vi "Register for gRPC Server Events.vi"(8 "error in (no error)":errorcluster, 11 "Plugin Manager in":refnum<class "CIFPluginManager.lvclass">) -> (0 "error out":errorcluster, 2 "Event Registration Refnum":refnum<event-registration>, 3 "Plugin Manager out":refnum<class "CIFPluginManager.lvclass">)   [LabVIEW 2021, in "CIFPluginManager.lvclass"]
uses:
  CIFPluginManager.lvclass
  CIF_Manager_server/RPC Service/Manager/Manager.lvclass
  C:/Program Files/National Instruments/LabVIEW 2021/vi.lib/gRPC/LabVIEW gRPC Servicer/ServiceBase/ServiceBase.lvclass
  CIF_Manager_server/RPC Service/Manager/Manager.lvclass/Manager.ctl
  CIFPluginManager.lvclass/CIFPluginManager.ctl
  D:/dev/CIF-LVCore/src/CIFPluginManager/CIFPluginManager/gRPC/CIF_Manager_server/RPC Service/Manager/Manager.lvclass
  <vilib>/gRPC/LabVIEW gRPC Library/Shared/grpcId.ctl
  <vilib>/gRPC/LabVIEW gRPC Library/grpc-lvsupport-release.lvlib
  <vilib>/gRPC/LabVIEW gRPC Library/Server API/typeDefs/gRPCId Cluster.ctl
  CIF_Manager_server/RPC Service/Manager/typeDefs/Server gRPC UEs.ctl
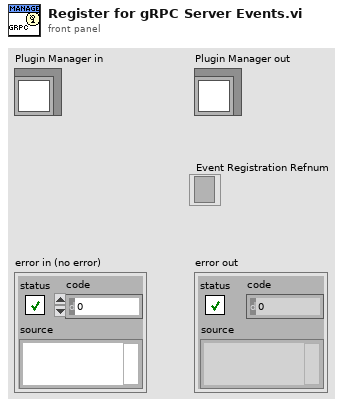
[diagram p1: front panel]
types:
  T1 = typedef "CIF_Manager_server.lvlib/Manager.lvclass/Server gRPC UEs.ctl" = cluster{"Manager LoadPlugin gRPC UE":refnum<user-event>, "Manager RegisterPlugin gRPC UE":refnum<user-event>, "Manager UnregisterPlugin gRPC UE":refnum<user-event>, "Manager QueryPluginTypes gRPC UE":refnum<user-event>, "Manager AbortPlugin gRPC UE":refnum<user-event>, "Manager UnloadAllPlugins gRPC UE":refnum<user-event>, "Manager Destroy gRPC UE":refnum<user-event>, "Manager Ping gRPC UE":refnum<user-event>, "Manager QueryErrors gRPC UE":refnum<user-event>, "Manager QueryConfig gRPC UE":refnum<user-event>, "Manager QueryInfo gRPC UE":refnum<user-event>, "Manager ResetErrorIndex gRPC UE":refnum<user-event>, "Manager ResetConfigIndex gRPC UE":refnum<user-event>, "Manager ResetInfoIndex gRPC UE":refnum<user-event>, "Manager QueryPluginInfo gRPC UE":refnum<user-event>, "Manager QueryPlugin gRPC UE":refnum<user-event>, "Manager QuerySystemStatus gRPC UE":refnum<user-event>, "Manager UpdateClock gRPC UE":refnum<user-event>, "Manager CreateOrch gRPC UE":refnum<user-event>, "Manager QueryClockStatus gRPC UE":refnum<user-event>, "Manager QueryAllChannels gRPC UE":refnum<user-event>, "Manager RegisterPluginLoader gRPC UE":refnum<user-event>, "Manager CreatePluginLoader gRPC UE":refnum<user-event>, "Manager DestroyPluginLoader gRPC UE":refnum<user-event>}
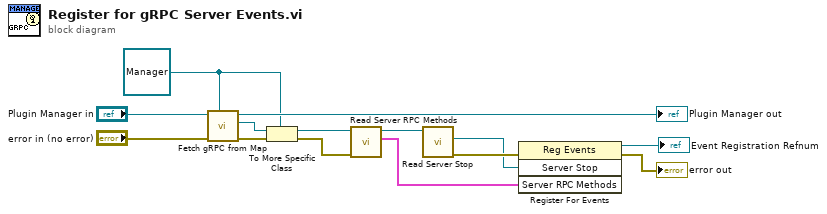
[diagram p0: block diagram]
diagram:
  w11 = refnum<class "Manager.lvclass"> refnum ("CIF_Manager_server.lvlib:Manager.lvclass")
  n1 = call "Fetch gRPC from Map.vi"("gRPC Server Class type"=w11, "error in (no error)"="error in (no error)", "Plugin Manager in"="Plugin Manager in") -> ("error out"=w10:errorcluster, "gRPC Server Class out"=w12:refnum<class "ServiceBase.lvclass">, "Plugin Manager out"=→"Plugin Manager out":refnum<class "CIFPluginManager.lvclass">)  [unwired: 6 in]
  n2 = To More Specific Class(target class=w11, reference=w12, error in=w10) -> (specific class reference=w4:refnum<class "Manager.lvclass">, error out=w8:errorcluster)
  n3 = call "Read Server RPC Methods.vi"("error in (no error)"=w8, "SignalGeneratorService in"=w4) -> ("Server RPC Methods"=w5:T1, "SignalGeneratorService out"=w13:refnum<class "Manager.lvclass">)  [unwired: 7 in, 1 out]
  n4 = call-dynamic "Read Server Stop.vi"("iService in"=w13) -> ("error out"=w7:errorcluster, "Server Stop"=w6:refnum<user-event>)  [unwired: 8 in, 1 out]
  n5 = register-events(error in=w7, w6, w5) -> (reference out=→"Event Registration Refnum":refnum<event-registration>, error out=→"error out":errorcluster)  [unwired: 1 in]
